vi "GoTo para tangente.vi"(6 "Reinitialize":bool, 10 "Target":dbl[](array[numeric]), 11 "Position":dbl[](array[numeric])) -> (0 "errors":dbl[](array[numeric]), 3 "Output\nVelocity":dbl[](array[numeric]) format="%.2f")   [LabVIEW 2016]
uses:
  <vilib>/Analysis/coordinate.llb/2D Cartesian Coordinate Rotation (Scalar).vi
  <vilib>/addons/control/pid/pid.llb/PID (DBL Array).vi
  <vilib>/addons/control/pid/NI_PID_pid.lvlib
  <vilib>/Analysis/NI_AALPro.lvlib
panel:
  in  "output range":cluster{"output high":dbl, "output low":dbl}[](array[cluster])=[{"output high"=0.88, "output low"=-0.88}, {"output high"=0.88, "output low"=-0.88}, {"output high"=1.0, "output low"=-1.0}]
  in  "PID gains":T1(array[cluster])=[{"proportional gain (Kc)"=0.0012, "integral time (Ti, min)"=0.0, "derivative time (Td, min)"=0.0}, {"proportional gain (Kc)"=1.5, "integral time (Ti, min)"=0.0, "derivative time (Td, min)"=0.0}]
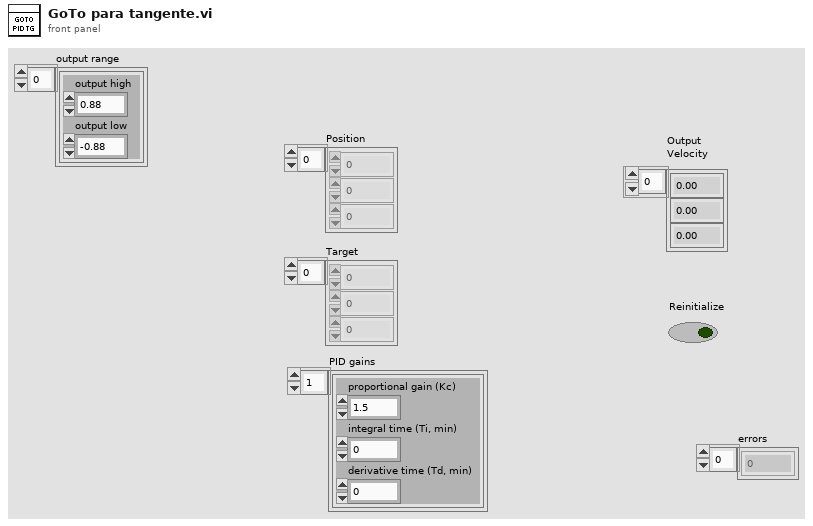
[diagram p1: front panel]
types:
  T1 = cluster{"proportional gain (Kc)":dbl, "integral time (Ti, min)":dbl, "derivative time (Td, min)":dbl}[]
  T2 = cluster{"proportional gain (Kc)":dbl, "integral time (Ti, min)":dbl, "derivative time (Td, min)":dbl}
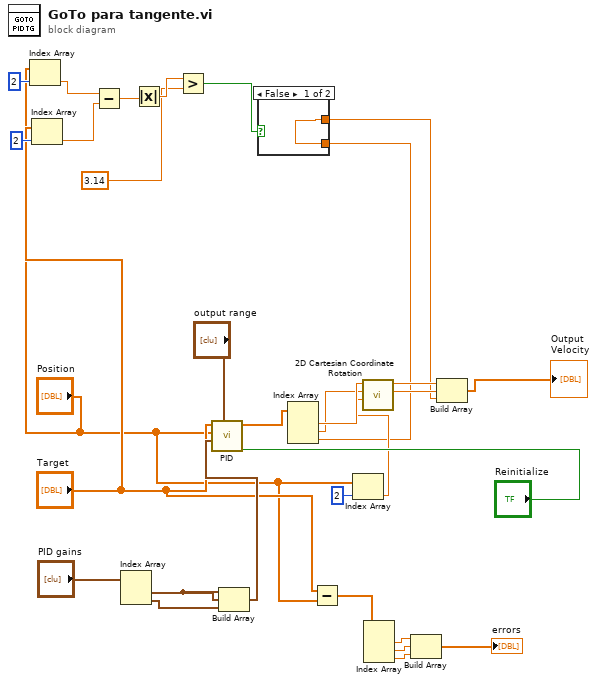
[diagram p0: block diagram]
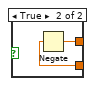
[diagram p2: hidden frame]
diagram:
  n1 = Index Array(array="Position", index=2) -> (element=w15:dbl)
  n2 = Index Array(array="Target", index=2) -> (element=w14:dbl)
  n3 = Subtract(x=w15, y=w14) -> (x-y=w13:dbl)
  n4 = Index Array(array="PID gains") -> (element #1=w20:T2, element #2=w19:T2)  [unwired: 2 in]
  n5 = Absolute Value(x=w13) -> (abs(x)=w12:dbl)
  n6 = Greater?(x=w12, y=3.14) -> (0:w10:bool)
  n7 = Build Array(w20, w20, w19) -> (w18:T1)
  n8 = call-poly <vilib>:"PID.vi"("reinitialize? (F)"="Reinitialize", "output range"="output range", "PID gains"=w18, "process variable"="Position", "setpoint"="Target") -> ("output"=w29:dbl[])  [unwired: 5 in, 1 out]
  n9 = Index Array(array=w29) -> (element #1=w28:dbl, element #2=w27:dbl, element #3=w9:dbl)  [unwired: 3 in]
  n10 = case shown="False" w10 {
    tunnel: w9 -> [w32 w34]
    tunnel: [w32 w33] -> w8
    frame False {
    }
    frame True {
      n11 = Negate(x=w34) -> (-x=w33:dbl)
    }
  }
  n12 = Subtract(x="Target", y="Position") -> (x-y=w5:dbl[])
  n13 = Index Array(array="Position", index=2) -> (element=w22:dbl)
  n14 = call-poly <vilib>:"2D Cartesian Coordinate Rotation.vi"("theta"=w22, "y"=w27, "x"=w28) -> ("y out"=w25:dbl, "x out"=w26:dbl)  [unwired: 6 in, 1 out]
  n15 = Index Array(array=w5) -> (element #1=w4:dbl, element #2=w3:dbl, element #3=w2:dbl)  [unwired: 3 in]
  n16 = Build Array(w4, w3, w2) -> (→"errors":dbl[])
  n17 = Build Array(w26, w25, w8) -> (→"Output\nVelocity":dbl[])
